vi "KE622x -- Get RS-232 Params.vi"(0 "Resource In":refnum<visa-resource-name>, 1 "Check For SCPI Errors? (T)":bool=TRUE, 11 "error in (no error)":errorcluster, 12 "Term Char (0xA)":u8=10 format="%02x") -> (4 "Resource Out (dupl)":refnum<visa-resource-name>, 15 "error out":errorcluster)   [LabVIEW 2019, in "Keithley 622x.lvlib"]
uses:
  Keithley 622x.lvlib
  Typedefs/KE622x -- Serial Port Settings.ctl
panel:
  out "RS-232 Settings":T1={"Read Term Char"=enum."CR", "Baud Rate"=enum."19200", "Flow Control\n(XON / XOFF)"=enum."Off"}
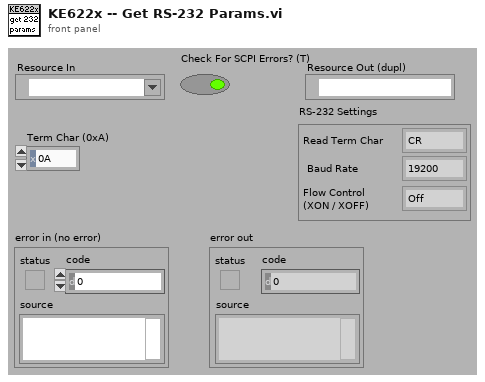
[diagram p1: front panel]
types:
  T1 = typedef "Keithley 622x.lvlib/KE622x -- Serial Port Settings.ctl" = cluster{"Read Term Char":enum16{"CR", "LF", "CR + LF", "LF + CR"}, "Baud Rate":enum16{"300", "600", "1200", "2400", "4800", "9600", "19200", "38400", "57600", "115200"}, "Flow Control\n(XON / XOFF)":enum16{"Off", "On"}}
  T2 = enum16{"300", "600", "1200", "2400", "4800", "9600", "19200", "38400", "57600", "115200"}
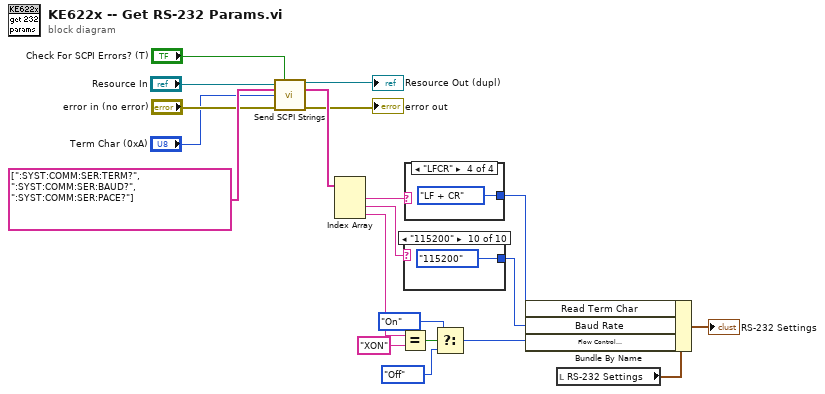
[diagram p0: block diagram]
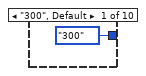
[diagram p2: hidden frame]
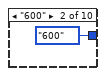
[diagram p3: hidden frame]
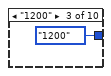
[diagram p4: hidden frame]
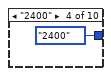
[diagram p5: hidden frame]
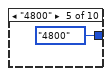
[diagram p6: hidden frame]
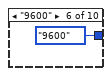
[diagram p7: hidden frame]
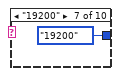
[diagram p8: hidden frame]
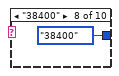
[diagram p9: hidden frame]
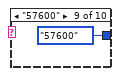
[diagram p10: hidden frame]
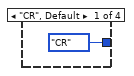
[diagram p11: hidden frame]
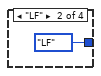
[diagram p12: hidden frame]
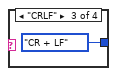
[diagram p13: hidden frame]
diagram:
  n1 = call "Send SCPI Strings.vi"("Resource In"="Resource In", "Check For SCPI Errors? (T)"="Check For SCPI Errors? (T)", "SCPI Strings (no term char)"=string[] [":SYST:COMM:SER:TERM?", ":SYST:COMM:SER:BAUD?", ":SYST:COMM:SER:PACE?"], "Term Char (0xA)"="Term Char (0xA)", "error in (no error)"="error in (no error)") -> ("Resource Out (dupl)"=→"Resource Out (dupl)":refnum<visa-resource-name>, "Query Responses"=w16:string[], "error out"=→"error out":errorcluster)  [unwired: 7 in, 1 out]
  n2 = Index Array(array=w16) -> (element #1=w15:string, element #2=w13:string, element #3=w12:string)  [unwired: 3 in]
  n3 = Equal?(x=w12, y="XON") -> (x = y?=w9:bool)
  n4 = case shown="\"115200\"" w13 {
    tunnel: [T2."300" ("Baud Rate") T2."600" ("Baud Rate") T2."1200" ("Baud Rate") T2."2400" ("Baud Rate") T2."4800" ("Baud Rate") T2."9600" ("Baud Rate") T2."19200" ("Baud Rate") T2."38400" ("Baud Rate") T2."57600" ("Baud Rate") T2."115200" ("Baud Rate")] -> w3
    frame "300", Default {
    }
    frame "600" {
    }
    frame "1200" {
    }
    frame "2400" {
    }
    frame "4800" {
    }
    frame "9600" {
    }
    frame "19200" {
    }
    frame "38400" {
    }
    frame "57600" {
    }
    frame "115200" {
    }
  }
  n5 = case shown="\"LFCR\"" w15 {
    tunnel: [enum16{"CR", "LF", "CR + LF", "LF + CR"}."CR" ("Term Char") enum16{"CR", "LF", "CR + LF", "LF + CR"}."LF" ("Term Char") enum16{"CR", "LF", "CR + LF", "LF + CR"}."CR + LF" ("Term Char") enum16{"CR", "LF", "CR + LF", "LF + CR"}."LF + CR" ("Term Char")] -> w10
    frame "CR", Default {
    }
    frame "LF" {
    }
    frame "CRLF" {
    }
    frame "LFCR" {
    }
  }
  n6 = Select(t=enum16{"Off", "On"}."On", s=w9, f=enum16{"Off", "On"}."Off" ("Flow Control\n(XON / XOFF)")) -> (s? t:f=w6:enum16{"Off", "On"})
  n7 = local read "RS-232 Settings"() -> (w14:T1)
  n8 = Bundle By Name(cluster=w14, "Read Term Char"=w10, "Baud Rate"=w3, "Flow Control\n(XON / XOFF)"=w6) -> (→"RS-232 Settings":T1)
